vi "test_polymophic.vi"() -> ()   [LabVIEW 2020]
uses:
  API/Create From VI Reference.vi
  API/Destroy.vi
  CSM-Helper.lvclass
panel:
  out "error out":errorcluster
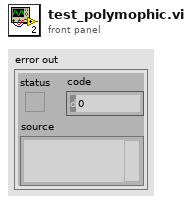
[diagram p1: front panel]
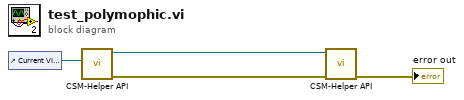
[diagram p0: block diagram]
diagram:
  n1 = control-ref of="Current VI Reference"() -> (w2:refnum<vi>)
  n2 = call-poly "CSM-Helper API.vi"("VI"=w2) -> ("error out"=w4:errorcluster, "CSM-Helper.lvclass"=w3:refnum<class "CSM-Helper.lvclass">)  [unwired: 9 in]
  n3 = call-poly "CSM-Helper API.vi"("error in (no error)"=w4, "CSM-Helper in"=w3) -> ("error out"=→"error out":errorcluster)  [unwired: 8 in, 1 out]
